vi "Newton_P(x0) & P'(x0).vi"(10 "x0":dbl, 11 "P(x)":dbl[](array[numeric])) -> (2 "P'(x0)":dbl, 3 "P(x0)":dbl)   [LabVIEW 2017, in "NI_AALPro.lvlib"]
uses:
  <vilib>/Analysis/NI_AALPro.lvlib
  <vilib>/Analysis/polynomials.llb/Scalar Polynomial Evaluation (DBL).vi
  <vilib>/Analysis/polynomials.llb/nth Derivative of Polynomial (DBL).vi
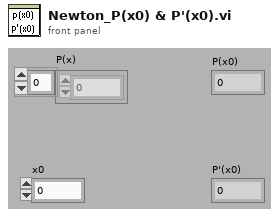
[diagram p1: front panel]
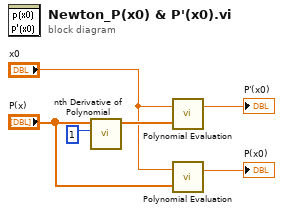
[diagram p0: block diagram]
diagram:
  n1 = call-poly <vilib>:"nth Derivative of Polynomial.vi"("order"=1, "P(x)"="P(x)") -> ("Nth Derivative of P(x)"=w5:dbl[])  [unwired: 8 in, 1 out]
  n2 = call-poly <vilib>:"Polynomial Evaluation.vi"("P(x)"=w5, "a"="x0") -> ("P(a)"=→"P'(x0)":dbl)  [unwired: 1 out]
  n3 = call-poly <vilib>:"Polynomial Evaluation.vi"("P(x)"="P(x)", "a"="x0") -> ("P(a)"=→"P(x0)":dbl)  [unwired: 1 out]
